vi "Send Recieve Acknowledge Initialized.vi"(7 "Message Priority (Normal)":T1=enum."Normal", 8 "error in (no error)":errorcluster, 9 "Requestor":string, 10 "Requestee":string, 11 "Message Enqueuer":refnum<class "Message Enqueuer.lvclass">) -> (0 "error out":errorcluster, 3 "Message Enqueuer out":refnum<class "Message Enqueuer.lvclass">)   [LabVIEW 2015, in "Recieve Acknowledge Initialized Msg.lvclass"]
doc: "This VI sends the message to an actor."
uses:
  Recieve Acknowledge Initialized Msg.lvclass
  <vilib>/ActorFramework/Message Enqueuer/Message Enqueuer.lvclass
  <vilib>/ActorFramework/Message Enqueuer/Message Priority.ctl
  Recieve Acknowledge Initialized Msg.lvclass/Recieve Acknowledge Initialized Msg.ctl
  <vilib>/ActorFramework/Message Enqueuer/Message Enqueuer.lvclass/Message Enqueuer.ctl
  <vilib>/ActorFramework/Message Priority Queue/Priority Enqueue.vi
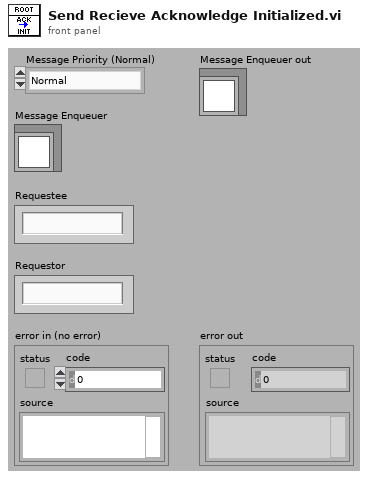
[diagram p1: front panel]
types:
  T1 = typedef "Actor Framework.lvlib/Message Enqueuer.lvclass/Message Priority.ctl" = enum16{"Low", "Normal", "High"}
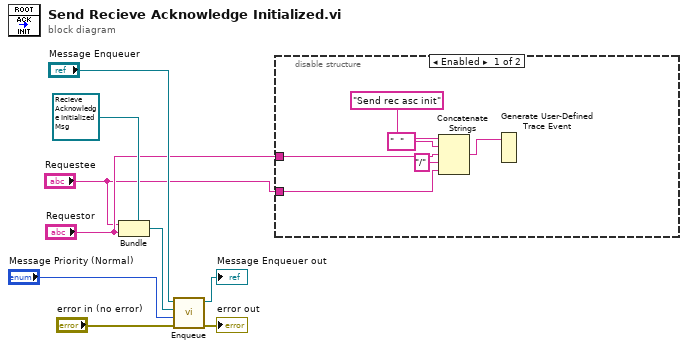
[diagram p0: block diagram]
diagram:
  n1 = Bundle(cluster=refnum<class "Recieve Acknowledge Initialized Msg.lvclass"> refnum ("Object"), "Requestee", "Requestor") -> (w5:refnum<class "Recieve Acknowledge Initialized Msg.lvclass">)
  n2 = call <vilib>:"Enqueue.vi"("error in (no error)"="error in (no error)", "Message Priority (Normal)"="Message Priority (Normal)", "Message"=w5, "Message Enqueuer in"="Message Enqueuer") -> ("error out"=→"error out":errorcluster, "Message Enqueuer out"=→"Message Enqueuer out":refnum<class "Message Enqueuer.lvclass">)  [unwired: 6 in]
  n3 = disable-structure shown="Enabled" {
    disable-tunnel: "Requestee" -> [w11 _]
    disable-tunnel: "Requestor" -> [w14 _]
    frame Enabled {
      n4 = Concatenate Strings("Send rec asc init" ("string"), "  " ("string"), w14, "/" ("string"), w11) -> (w10:string)
      n5 = Generate User-Defined Trace Event(2:w10) -> ()  [unwired: 1 in]
    }
    frame Disabled {
    }
  }
